vi "ConfigureAcquisition.vi"(8 "error in (no error)":errorcluster, 11 "IVI_Class in":refnum<class "IVI_Class.lvclass">) -> (0 "error out":errorcluster, 3 "IVI_Class out":refnum<class "IVI_Class.lvclass">)   [LabVIEW 2018, in "ScopePlugins.lvlib" / "IVI_Class.lvclass"]
uses:
  IVI_Class.lvclass
  C:/Users/ico/Documents/Projects/NistPluggableModules/Scope/ScopePlugins/ScopePluginBaseClass/ScopePluginsBase.lvclass
  ScopePluginBaseClass/ScopePluginsBase.lvclass/ScopePluginsBase.ctl
  ScopePluginBaseClass/Accessors/Read Channels.vi
  ScopePluginBaseClass/Accessors/Read Handle.vi
  <vilib>/Utility/error.llb/Error Cluster From Error Code.vi
  <vilib>/ErrorRing/Error Ring.xnode
  ScopePluginBaseClass/ScopePluginsBase.lvclass
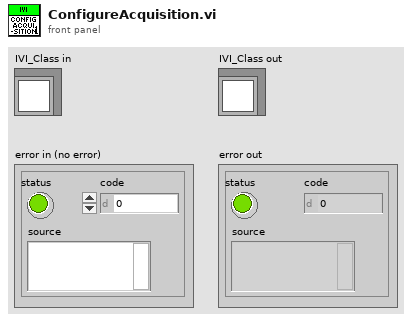
[diagram p1: front panel]
types:
  T1 = enum16{"Normal", "PeakDetect", "HighRes", "Envelope", "Average"}
  T2 = typedef "ScopePlugins.lvlib/ScopePluginsBase.lvclass/ChannelSetting(s).ctl" = cluster{"Number of Channels":i32, "Channel(s)":cluster{"Enabled":bool, "Instrument Handle":string, "Channel Name":string, "Maximum Input Frequency":dbl, "Verticle Settings":cluster{"Vertical Range":dbl, "Vertical Offset":dbl, "Probe Attenuation":dbl, "Vertical Coupling":i32}, "Connected":bool, "Input Impedance":dbl}[]}
  T3 = typedef "ScopePlugins.lvlib/ScopePluginsBase.lvclass/HorizontalSettings.ctl" = cluster{"Continuous":bool, "EnableAveraging":bool, "Number Averages":i32, "Measurement Timeout":dbl, "Min Record Length":i32, "Min Sample Rate":dbl, "Enforce Realtime":bool, "Sampling Mode ":enum16{"Real Time", "Equivalent Time", "Segment", "Real Time Peak Detect", "Real Time High Resolution", "Peak Detect Segment", "High Resolution Segment"}, "Interpolation":enum16{"No Interpolation", "sin(x)/x", "linear", "1 Point sin(x)/x", "2 Point sin(x)/x", "4 Point sin(x)/x", "8 Point sin(x)/x", "16 Point sin(x)/x"}, "Type":enum16{"Normal", "PeakDetect", "HighRes", "Envelope", "Average"}, "StartTime":dbl, "Time Per Record":dbl, "Number of Points Minimum":i32}
  T4 = cluster{"Enabled":bool, "Instrument Handle":string, "Channel Name":string, "Maximum Input Frequency":dbl, "Verticle Settings":cluster{"Vertical Range":dbl, "Vertical Offset":dbl, "Probe Attenuation":dbl, "Vertical Coupling":i32}, "Connected":bool, "Input Impedance":dbl}[]
  T5 = enum16{"No Interpolation", "sin(x)/x", "linear", "1 Point sin(x)/x", "2 Point sin(x)/x", "4 Point sin(x)/x", "8 Point sin(x)/x", "16 Point sin(x)/x"}
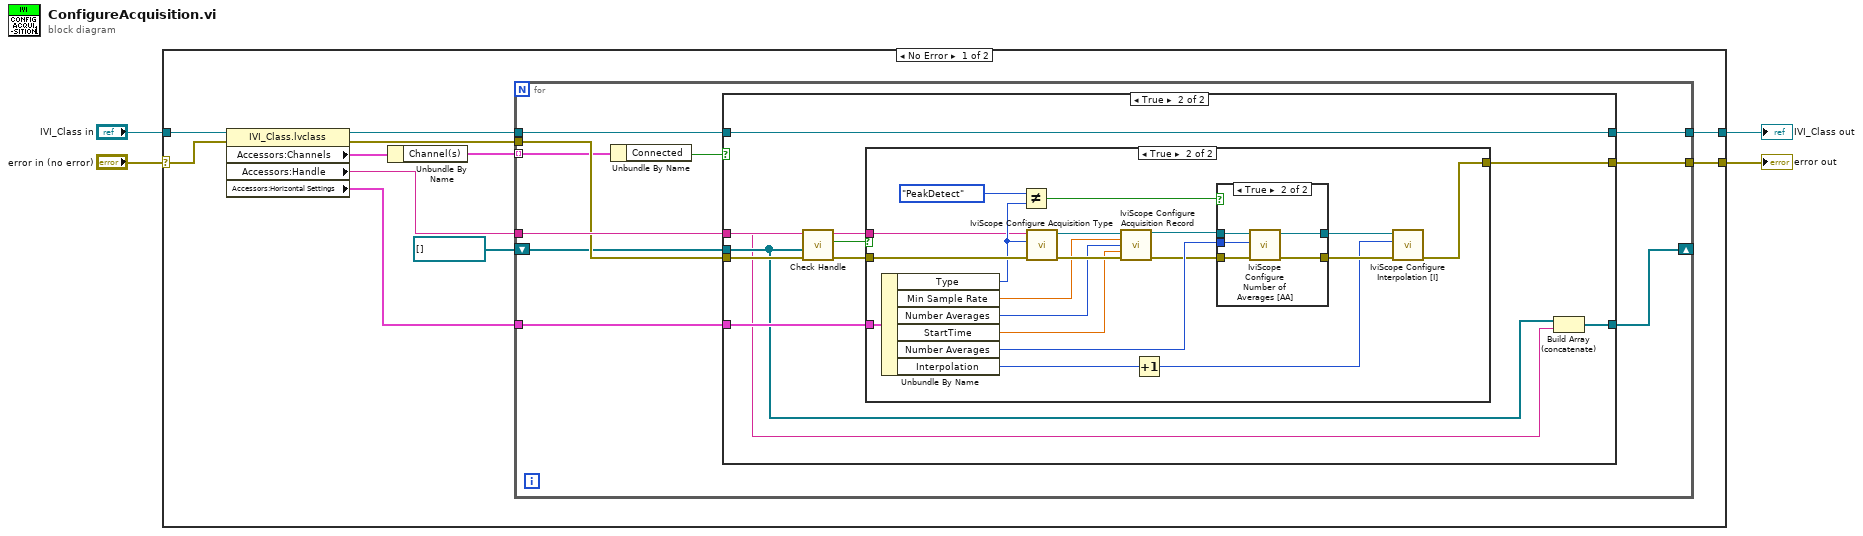
[diagram p0: block diagram]
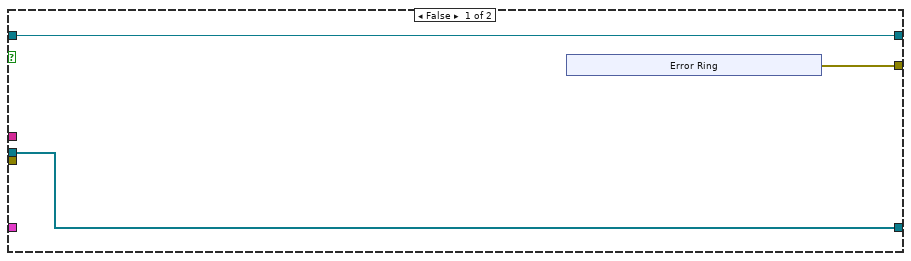
[diagram p2: hidden frame]
diagram:
  n1 = case shown="No Error" "error in (no error)" {
    selector: "error in (no error)" -> [w14 w71]
    tunnel: "IVI_Class in" -> [w15 w72]
    tunnel: [w11 w72] -> w2
    tunnel: [w12 w71] -> w1
    frame No Error {
      n2 = property class="IVI_Class.lvclass"(reference=w15, error in=w14) -> (reference out=w13:refnum<class "IVI_Class.lvclass">, error out=w10:errorcluster, "Accessors:Channels"=w9:T2, "Accessors:Handle"=w7:string, "Accessors:Horizontal Settings"=w5:T3)
      n3 = Unbundle By Name(w9) -> ("Channel(s)"=w8:T4)
      n4 = for {
        tunnel: [w24] -> w12
        tunnel: w10 -> [w20]
        tunnel: w8 -> [w19] mode=indexing
        tunnel: w13 -> [w25]
        tunnel: [w23] -> w11
        tunnel: w7 -> [w21]
        shift-right: [w16] -> _
        shift-left: refnum<k15>[] [] -> [w17]
        tunnel: w5 -> [w18]
        n5 = Unbundle By Name(w19) -> ("Connected"=w22:bool)
        n6 = case shown="True" w22 {
          tunnel: w25 -> [w28 w43]
          tunnel: [w27 w42] -> w24
          tunnel: [w28 w43] -> w23
          tunnel: w20 -> [_ w40]
          tunnel: w21 -> [_ w39]
          tunnel: w18 -> [_ w41]
          tunnel: w17 -> [w26 w37]
          tunnel: [w26 w35] -> w16
          frame False {
            n7 = xnode "Error Ring"() -> ("error out"=w27:errorcluster)
          }
          frame True {
            n8 = call "Check Handle.vi"("error in (no error)"=w40, "Array"=w37, "Handle In"=w39) -> ("error out"=w38:errorcluster, "Duplicate Instrument?"=w34:bool, "Handle Out"=w36:string)  [unwired: 6 in]
            n9 = case shown="True" w34 {
              tunnel: [w44 w53] -> w42
              tunnel: w41 -> [_ w48]
              tunnel: w38 -> [w44 w47]
              tunnel: w36 -> [_ w45]
              frame False {
              }
              frame True {
                n10 = Unbundle By Name(w48) -> ("Type"=w46:T1, "Min Sample Rate"=w61:dbl, "Number Averages"=w60:i32, "StartTime"=w59:dbl, "Number Averages"=w58:i32, "Interpolation"=w51:T5)
                n11 = Not Equal?(x=T1."PeakDetect" ("y"), y=w46) -> (x != y?=w49:bool)
                n12 = call <vilib>:"IviScope Configure Acquisition Type.vi"("error in (no error)"=w47, "acquisition type (Normal)"=w46, "instrument handle"=w45) -> ("error out"=w62:errorcluster, "instrument handle out"=w63:refnum<k15>)  [unwired: 7 in]
                n13 = call <vilib>:"IviScope Configure Acquisition Record.vi"("instrument handle"=w63, "time per record (1.0E-3 s)"=w61, "min record length (100 samples)"=w60, "acquisition start time (0.0 s)"=w59, "error in (no error)"=w62) -> ("instrument handle out"=w57:refnum<k15>, "error out"=w56:errorcluster)  [unwired: 9 in]
                n14 = Increment(x=w51) -> (x+1=w52:T5)
                n15 = case shown="True" w49 {
                  tunnel: w58 -> [_ w70]
                  tunnel: w57 -> [w65 w69]
                  tunnel: w56 -> [w64 w68]
                  tunnel: [w65 w67] -> w55
                  tunnel: [w64 w66] -> w54
                  frame False {
                  }
                  frame True {
                    n16 = call <vilib>:"IviScope Configure Number of Averages [AA].vi"("error in (no error)"=w68, "number of averages (8)"=w70, "instrument handle"=w69) -> ("error out"=w66:errorcluster, "instrument handle out"=w67:refnum<k15>)  [unwired: 7 in]
                  }
                }
                n17 = call <vilib>:"IviScope Configure Interpolation [I].vi"("error in (no error)"=w54, "interpolation"=w52, "instrument handle"=w55) -> ("error out"=w53:errorcluster)  [unwired: 7 in, 1 out]
              }
            }
            n18 = Build Array (concatenate)(w37, w36) -> (w35:refnum<k15>[])
          }
        }
      }
    }
    frame Error {
    }
  }
  "error out" <- w1
  "IVI_Class out" <- w2
